vi "质控内部交互全局.vi"() -> ()   [LabVIEW 2016, in "质控单元.lvlib"]
panel:
  out "CODCr通讯状态":bool
  out "CODMn通讯状态":bool
  out "总氮通讯状态":bool
  out "总磷通讯状态":bool
  out "氨氮通讯状态":bool
  out "CODCr测量状态":u16[](array[numeric])
  out "CODMn测量状态":u16[](array[numeric])
  out "总氮测量状态":u16[](array[numeric])
  out "总磷测量状态":u16[](array[numeric])
  out "氨氮测量状态":u16[](array[numeric])
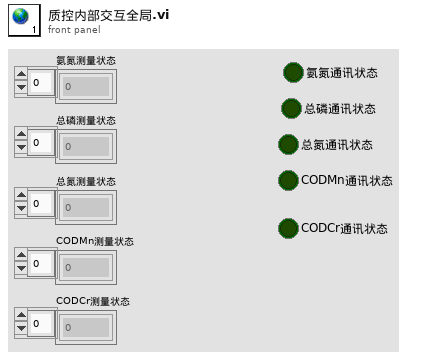
[diagram p1: front panel]
diagram:
